vi "engine version.vi"() -> (3 "Version":string="1.0.0.0")   [LabVIEW 2013, in "engine configuration.lvclass"]
uses:
  engine configuration.lvclass
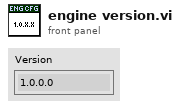
[diagram p1: front panel]
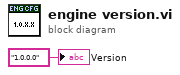
[diagram p0: block diagram]
diagram:
  "Version" <- "1.0.0.0" ("Version")
